vi "tester.vi"() -> ()   [LabVIEW 2020]
uses:
  <vilib>/Utility/miscctls.llb/LVSelectionTypeDef.ctl
panel:
  out "Diff":string
  out "Common String":string
  out "Missmatches 3":T1[](array[typedef])
  out "Common":string
  out "Missmatches 2":T1[](array[typedef])
  in  "Expected":string="Hello World!!"
  in  "Actual":string="Hey Anton!"
  in  "String":string
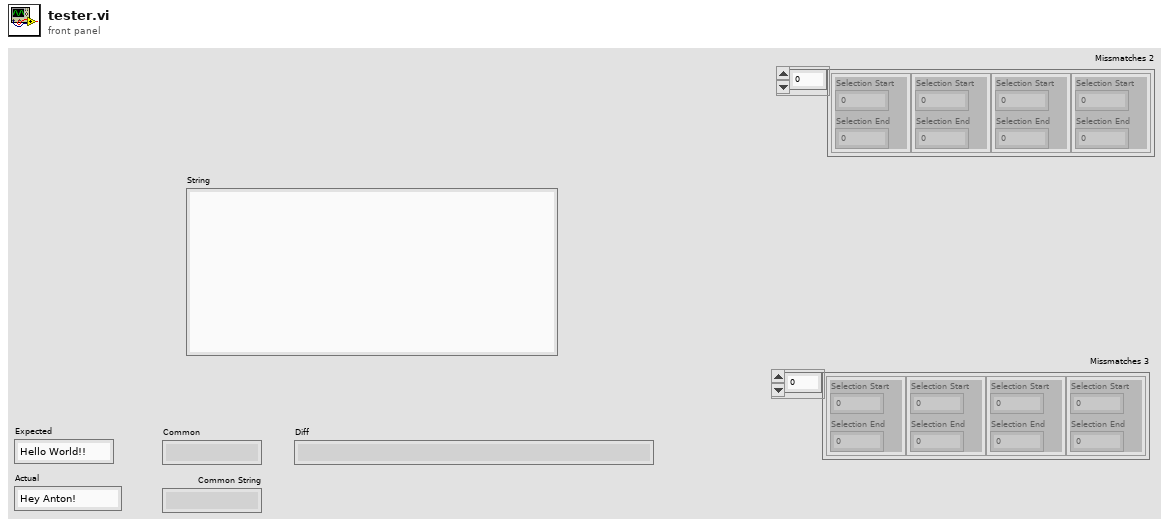
[diagram p1: front panel]
types:
  T1 = typedef "LVSelectionTypeDef.ctl" = cluster{"Selection Start":u32, "Selection End":u32}
  T2 = cluster{"Text.Selection":T1, "Text.Text Colors:Text Color":u32}[]
  T3 = cluster{"Selection Start":u32, "Selection End":u32}[]
  T4 = cluster{"Selection Start":u32, "Selection End":u32, "Type":enum16{"added", "missing"}}[]
  T5 = cluster{"Text.Selection":cluster{"Selection Start":u32, "Selection End":u32}, "Color":u32}
  T6 = cluster{"Text.Selection":cluster{"Selection Start":u32, "Selection End":u32}, "Text.Text Colors:Text Color":u32}
  T7 = cluster{"Selection Start":u32, "Selection End":u32}
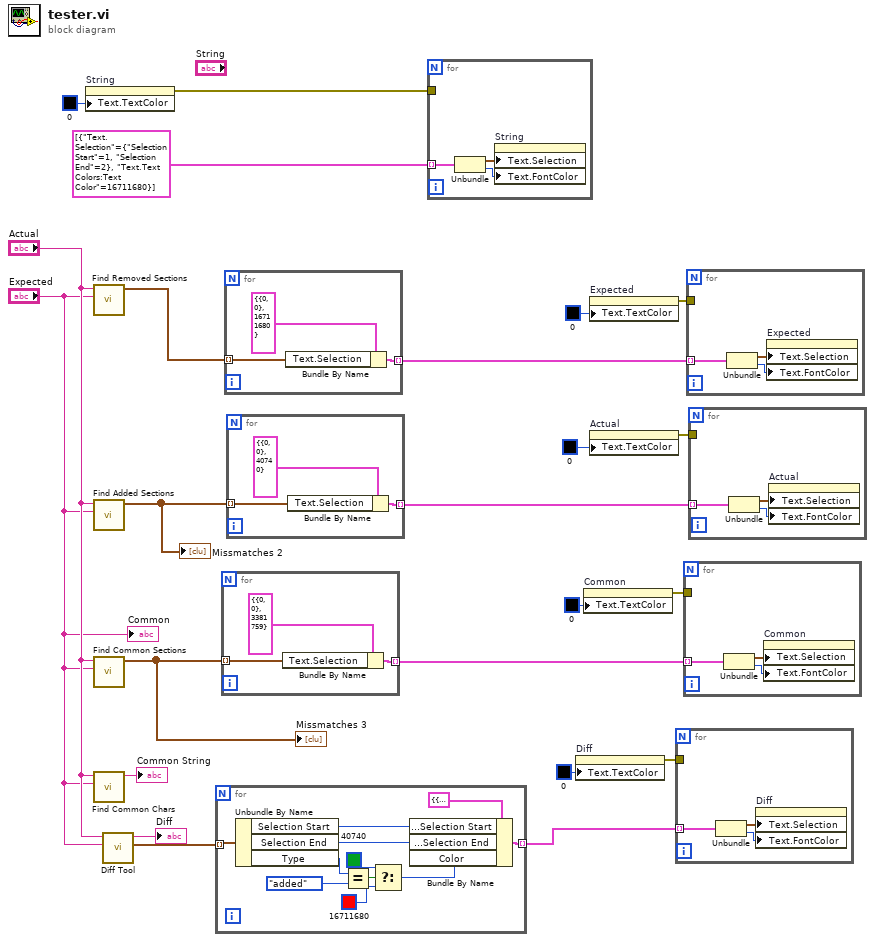
[diagram p0: block diagram]
diagram:
  n1 = property on="String" class="Str"("Text.TextColor"=u32 0 ("Text.Text Colors:Text Color")) -> (error out=w21:errorcluster)  [unwired: 2 in, 1 out]
  n2 = call "Find Removed Sections.vi"("Reference"="Expected", "Target"="Actual") -> ("Sections in Reference"=w13:T3)  [unwired: 9 in]
  n3 = call "Find Added Sections.vi"("Reference"="Expected", "Target"="Actual") -> ("Sections in Target"=w17:T3)  [unwired: 9 in]
  "Missmatches 2" <- w17
  n4 = call "Find Common Sections.vi"("Reference"="Expected", "Target"="Actual") -> ("Sections in Reference"=w12:T3)  [unwired: 9 in]
  "Missmatches 3" <- w12
  n5 = call "Find Common Chars.vi"("Reference"="Expected", "Target"="Actual") -> ("Common"=→"Common String":string)  [unwired: 9 in]
  n6 = call "Diff Tool.vi"("Reference"="Expected", "Target"="Actual") -> ("Highlights"=w2:T4, "Result"=→"Diff":string)  [unwired: 8 in]
  n7 = for {
    tunnel: w2 -> [w34] mode=indexing
    tunnel: [w28] -> w1 mode=indexing
    n8 = Unbundle By Name(w34) -> ("Selection Start"=w32:u32, "Selection End"=w31:u32, "Type"=w30:enum16{"added", "missing"})
    n9 = Equal?(x=w30, y=enum16{"added", "missing"}."added") -> (x = y?=w27:bool)
    n10 = Select(t=u32 40740 ("Text.Text Colors:Text Color"), s=w27, f=u32 16711680 ("Text.Text Colors:Text Color")) -> (s? t:f=w24:u32)
    n11 = Bundle By Name(cluster=T5 {"Text.Selection"={"Selection Start"=0, "Selection End"=0}, "Color"=40740} ("Colors"), "Text.Selection.Selection Start"=w32, "Text.Selection.Selection End"=w31, "Color"=w24) -> (w28:T5)
  }
  n12 = for {
    tunnel: w12 -> [w36] mode=indexing
    tunnel: [w35] -> w11 mode=indexing
    n13 = Bundle By Name(cluster=T6 {"Text.Selection"={"Selection Start"=0, "Selection End"=0}, "Text.Text Colors:Text Color"=3381759} ("Colors"), "Text.Selection"=w36) -> (w35:T6)
  }
  n14 = for {
    tunnel: w13 -> [w39] mode=indexing
    tunnel: [w38] -> w16 mode=indexing
    n15 = Bundle By Name(cluster=T6 {"Text.Selection"={"Selection Start"=0, "Selection End"=0}, "Text.Text Colors:Text Color"=16711680} ("Colors"), "Text.Selection"=w39) -> (w38:T6)
  }
  n16 = for {
    tunnel: w17 -> [w42] mode=indexing
    tunnel: [w41] -> w18 mode=indexing
    n17 = Bundle By Name(cluster=T6 {"Text.Selection"={"Selection Start"=0, "Selection End"=0}, "Text.Text Colors:Text Color"=40740} ("Colors"), "Text.Selection"=w42) -> (w41:T6)
  }
  n18 = for {
    tunnel: T2 [{"Text.Selection"={"Selection Start"=1, "Selection End"=2}, "Text.Text Colors:Text Color"=16711680}] ("Colors") -> [w46] mode=indexing
    tunnel: w21 -> [_]
    n19 = Unbundle(w46) -> ("Text.Selection"=w45:T1, "Text.Text Colors:Text Color"=w44:u32)
    n20 = property on="String" class="Str"("Text.Selection"=w45, "Text.FontColor"=w44) -> ()  [unwired: 2 in, 2 out]
  }
  n21 = property on="Diff" class="Str"("Text.TextColor"=u32 0 ("Text.Text Colors:Text Color")) -> (error out=w4:errorcluster)  [unwired: 2 in, 1 out]
  n22 = property on="Common" class="Str"("Text.TextColor"=u32 0 ("Text.Text Colors:Text Color")) -> (error out=w9:errorcluster)  [unwired: 2 in, 1 out]
  n23 = property on="Expected" class="Str"("Text.TextColor"=u32 0 ("Text.Text Colors:Text Color")) -> (error out=w14:errorcluster)  [unwired: 2 in, 1 out]
  n24 = property on="Actual" class="Str"("Text.TextColor"=u32 0 ("Text.Text Colors:Text Color")) -> (error out=w20:errorcluster)  [unwired: 2 in, 1 out]
  n25 = for {
    tunnel: w1 -> [w47] mode=indexing
    tunnel: w4 -> [_]
    n26 = Unbundle(w47) -> ("Text.Selection"=w49:T7, "Color"=w48:u32)
    n27 = property on="Diff" class="Str"("Text.Selection"=w49, "Text.FontColor"=w48) -> ()  [unwired: 2 in, 2 out]
  }
  n28 = for {
    tunnel: w11 -> [w50] mode=indexing
    tunnel: w9 -> [_]
    n29 = Unbundle(w50) -> ("Text.Selection"=w52:T7, "Text.Text Colors:Text Color"=w51:u32)
    n30 = property on="Common" class="Str"("Text.Selection"=w52, "Text.FontColor"=w51) -> ()  [unwired: 2 in, 2 out]
  }
  n31 = for {
    tunnel: w16 -> [w53] mode=indexing
    tunnel: w14 -> [_]
    n32 = Unbundle(w53) -> ("Text.Selection"=w55:T7, "Text.Text Colors:Text Color"=w54:u32)
    n33 = property on="Expected" class="Str"("Text.Selection"=w55, "Text.FontColor"=w54) -> ()  [unwired: 2 in, 2 out]
  }
  n34 = for {
    tunnel: w18 -> [w56] mode=indexing
    tunnel: w20 -> [_]
    n35 = Unbundle(w56) -> ("Text.Selection"=w58:T7, "Text.Text Colors:Text Color"=w57:u32)
    n36 = property on="Actual" class="Str"("Text.Selection"=w58, "Text.FontColor"=w57) -> ()  [unwired: 2 in, 2 out]
  }
  "Common" <- "Expected"
